vi "numeric_data.set.vi"(8 "error in (no error)":errorcluster, 10 "Numeric Data":i32[](array[numeric]), 11 "midi-file-event.meta in":refnum<class "midi-file-event.meta.lvclass">) -> (0 "error out":errorcluster, 3 "midi-file-event.meta out":refnum<class "midi-file-event.meta.lvclass">)   [LabVIEW 2020, in "midi-file-event.meta.lvclass"]
uses:
  midi-file-event.meta.lvclass
  midi-file-event.meta.lvclass/midi-file-event.meta.ctl
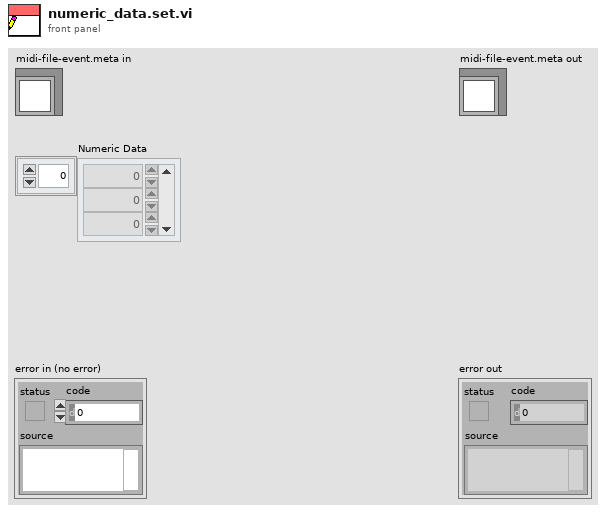
[diagram p1: front panel]
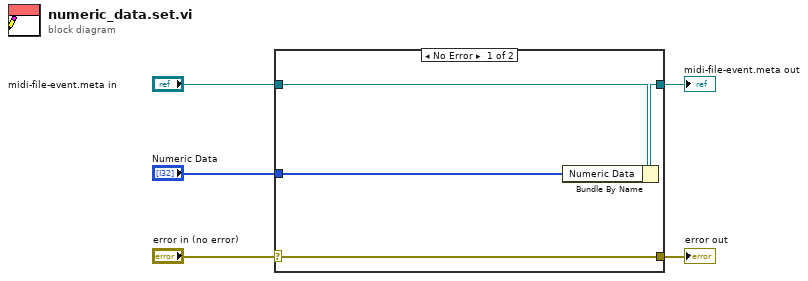
[diagram p0: block diagram]
diagram:
  n1 = case shown="No Error" "error in (no error)" {
    selector: "error in (no error)" -> [w9 w10]
    tunnel: [w9 w10] -> w4
    tunnel: [w7 w11] -> w2
    tunnel: "midi-file-event.meta in" -> [w8 w11]
    tunnel: "Numeric Data" -> [w6 _]
    frame No Error {
      n2 = Bundle By Name(cluster=w8, "Numeric Data"=w6) -> (w7:refnum<class "midi-file-event.meta.lvclass">)
    }
    frame Error {
    }
  }
  "error out" <- w4
  "midi-file-event.meta out" <- w2
